vi "ImgprocTest.vi"() -> ()   [LabVIEW 2012]
uses:
  <vilib>/vision/NI_Vision_Development_Module.lvlib
panel:
  in  "BCG Values (Brightness)":T1={"Brightness"=160.0, "Contrast"=50.0, "Gamma"=1.0}
  in  "Number of Erosion":i32=1
  out "Centroid (Centroid)":cluster{"X Centroid":sgl, "Y Centroid":sgl} {"Y Centroid" format="%.2f"; "X Centroid" format="%.2f"}
  out "Number of Particles":i32
  in  "Threshold":cluster{"Lower value":sgl, "Upper value":sgl}={"Lower value"=50.255474, "Upper value"=255.0} {"Upper value" scale=0.0..255.0; "Lower value" scale=0.0..255.0}
  out "Final":T2(plugin-control)
  out "Image":T2(plugin-control)
  out "Background":T2(plugin-control)
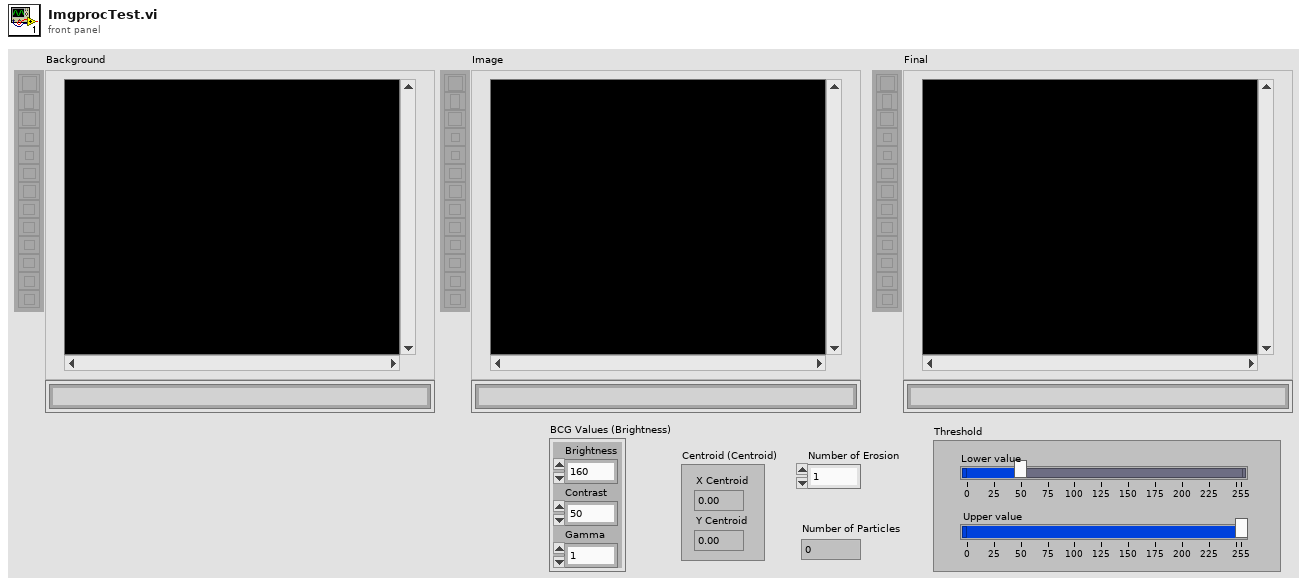
[diagram p1: front panel]
types:
  T1 = cluster{"Brightness":sgl, "Contrast":sgl, "Gamma":sgl}
  T2 = typedef "IMAQ Image.ctl" = refnum<image>
  T3 = typedef "Image Type" = u32
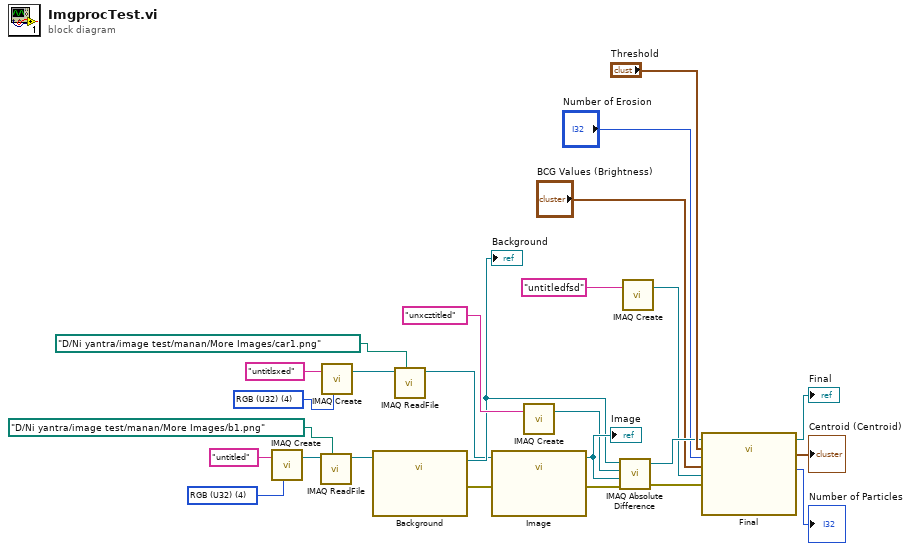
[diagram p0: block diagram]
diagram:
  w24 = T3 4 items=["Grayscale (U8)", "Grayscale (I16)", "Grayscale (SGL)", "Complex (CSG)", "RGB (U32)", "HSL (U32)", "RGB (U64)", "Grayscale (U16)"] ("Image Type")
  w25 = T3 4 items=["Grayscale (U8)", "Grayscale (I16)", "Grayscale (SGL)", "Complex (CSG)", "RGB (U32)", "HSL (U32)", "RGB (U64)", "Grayscale (U16)"] ("Image Type")
  n1 = call "IMAQ Create"("Image Name"="untitled", "Image Type"=w24) -> ("New Image"=w21:T2)  [unwired: 3 in, 1 out]
  n2 = call "IMAQ ReadFile"("File Path"=path "D:/Ni yantra/image test/manan/More Images/b1.png", "Image"=w21) -> ("Image Out"=w4:T2)  [unwired: 5 in, 4 out]
  n3 = call "IMAQ Create"("Image Name"="untitlsxed", "Image Type"=w25) -> ("New Image"=w20:T2)  [unwired: 3 in, 1 out]
  n4 = call "Background"("Image In"=w4) -> ("Image Out"=w10:T2, "error out"=w16:errorcluster)  [unwired: 25 in]
  "Background" <- w10
  n5 = call "IMAQ ReadFile"("File Path"=path "D:/Ni yantra/image test/manan/More Images/car1.png", "Image"=w20) -> ("Image Out"=w5:T2)  [unwired: 5 in, 4 out]
  n6 = call "Image"("Image In"=w5, "error in"=w16) -> ("Image Out"=w11:T2, "error out"=w15:errorcluster)  [unwired: 24 in]
  "Image" <- w11
  n7 = call "IMAQ Create"("Image Name"="unxcztitled") -> ("New Image"=w3:T2)  [unwired: 4 in, 1 out]
  n8 = call "IMAQ Absolute Difference"("Image Src A"=w10, "Image Dst"=w3, "Image Src B"=w11, "error in (no error)"=w15) -> ("Image Dst Out"=w7:T2, "error out"=w8:errorcluster)  [unwired: 3 in]
  n9 = call "IMAQ Create"("Image Name"="untitledfsd") -> ("New Image"=w6:T2)  [unwired: 4 in, 1 out]
  n10 = call "Final"("Image In"=w7, "Range (Threshold)"="Threshold", "Number of Erosion (Remove Particles)"="Number of Erosion", "BCG Values (Brightness)"="BCG Values (Brightness)", "Image Dst"=w6, "error in"=w8) -> ("Image Out"=→"Final":T2, "Centroid (Centroid)"=→"Centroid (Centroid)":cluster{"X Centroid":sgl, "Y Centroid":sgl}, "Number of Particles (Particle Analysis)"=→"Number of Particles":i32)  [unwired: 18 in, 1 out]
